vi "Folder Hierarchy to Tree.vi"(6 "Pattern":string, 8 "error in (no error)":errorcluster, 9 "Continue Recursing on Error? (F)":bool, 11 "File Explorer in":refnum<class "File Explorer.lvclass">) -> (0 "error out":errorcluster, 3 "File Explorer out":refnum<class "File Explorer.lvclass">)   [LabVIEW 2017, in "File Explorer.lvlib" / "File Explorer.lvclass"]
doc: "Parses the folder and harvests glyphs for each file type. Creates the tree items cluster for the tree control to render."
uses:
  <vilib>/gpm_packages/@cs/file-explorer-extension/Source/File Explorer/File Explorer/File Explorer.lvclass
  <vilib>/gpm_packages/@cs/file-explorer-extension/Source/File Explorer/File Explorer/File Explorer.lvclass/File Explorer.ctl
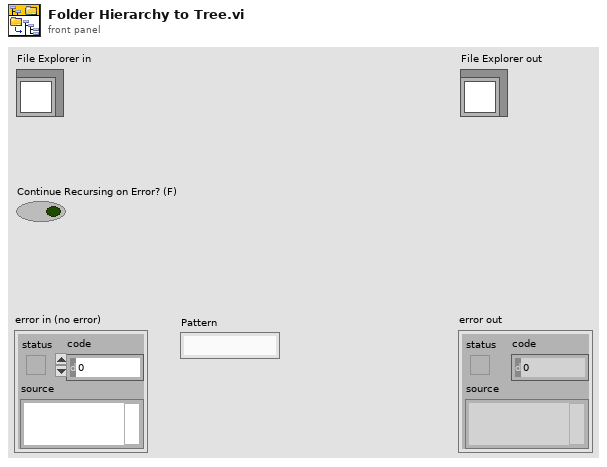
[diagram p1: front panel]
types:
  T1 = cluster{"Left Cell String":string, "Child Text":string[], "Child Tag":string, "Item Indent":i32, "Child Only?":bool, "Glyph Index":i32}
  T2 = typedef "imagedata.ctl" = cluster{"image type":i32, "image depth":i32, "image":u8[], "mask":u8[], "colors":u32[], "Rectangle":cluster{"left":i16, "top":i16, "right":i16, "bottom":i16}}
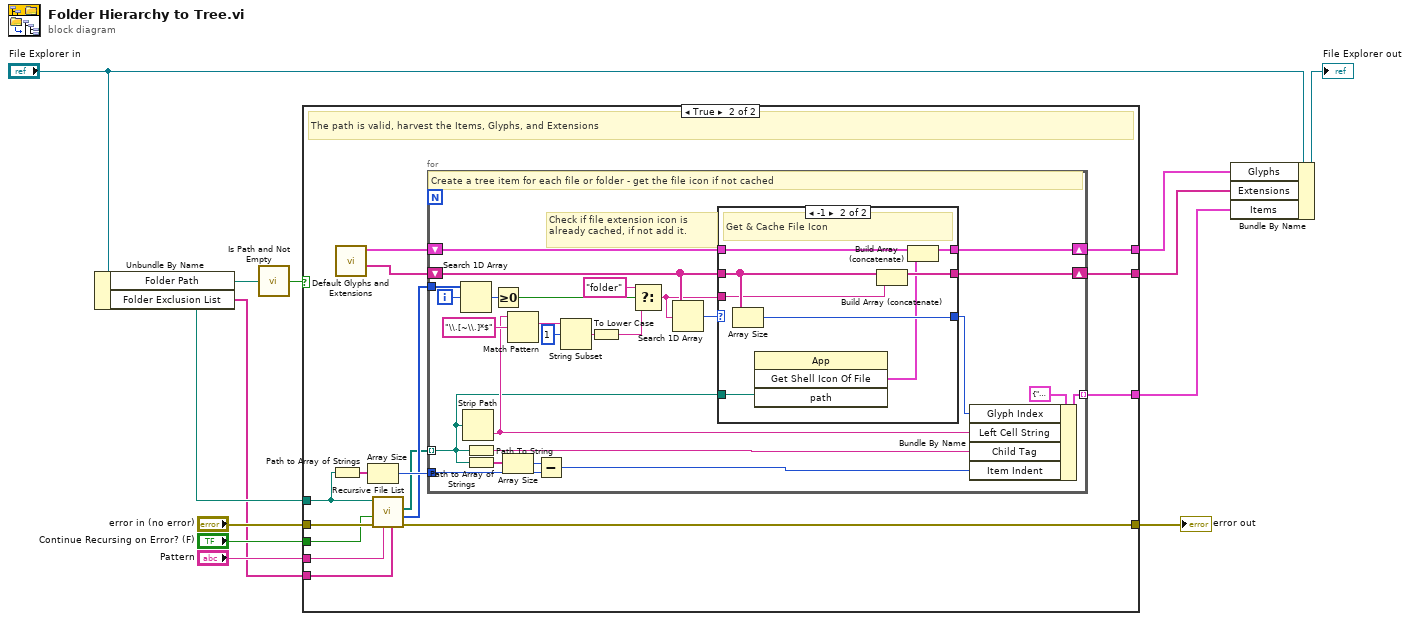
[diagram p0: block diagram]
diagram:
  n1 = Unbundle By Name("File Explorer in") -> ("Folder Path"=w7:path, "Folder Exclusion List"=w3:string[])
  n2 = call <vilib>:"Is Path and Not Empty.vi"("path"=w7) -> ("Is Path and Not Empty?"=w12:bool)  [unwired: 4 in]
  n3 = case shown="True" w12 {
    tunnel: w7 -> [_ w21]
    tunnel: [w13 w19] -> w10
    tunnel: "error in (no error)" -> [w13 w20]
    tunnel: "Continue Recursing on Error? (F)" -> [_ w16]
    tunnel: "Pattern" -> [_ w18]
    tunnel: w3 -> [_ w17]
    tunnel: [_ w26] -> w6
    tunnel: [_ w25] -> w5
    tunnel: [_ w24] -> w4
    frame False {
      # "The Path is either empty or Not a Path\nIn either case we will just ignore the request to recurse through the file hierarchy"
    }
    frame True {
      # "The path is valid, harvest the Items, Glyphs, and Extensions"
      n4 = Path to Array of Strings(0:w21) -> (2:w28:string[])  [unwired: 1 out]
      n5 = call <vilib>:"Default Glyphs and Extensions.vi"() -> ("Default Extensions"=w22:string[], "Default Glyphs"=w23:T2[])  [unwired: 10 in]
      n6 = Array Size(array=w28) -> (size(s)=w27:i32)
      n7 = call <vilib>:"Recursive File List.vi"("Folder to Exclude"=w17, "Pattern"=w18, "error in (no error)"=w20, "Continue Recursing on Error? (F)"=w16, "Folder Path"=w21) -> ("error out"=w19:errorcluster, "Folder Indexes"=w15:i32[], "Folders and Files"=w14:path[])  [unwired: 4 in]
      n8 = for {
        tunnel: w27 -> [w49]
        tunnel: w14 -> [w40] mode=indexing
        tunnel: [w48] -> w24 mode=indexing
        shift-right: [w37] -> w25
        shift-left: w22 -> [w36]
        shift-right: [w39] -> w26
        shift-left: w23 -> [w38]
        tunnel: w15 -> [w31]
        i -> [w32]
        # "Check if file extension icon is\nalready cached, if not add it."
        # "Create a tree item for each file or folder - get the file icon if not cached"
        n9 = Search 1D Array(1D array=w31, element=w32) -> (index of element=w30:i32)  [unwired: 1 in]
        n10 = Strip Path(path=w40) -> (name=w43:string)  [unwired: 1 out]
        n11 = Path To String(path=w40) -> (string=w53:string)
        n12 = Path to Array of Strings(0:w40) -> (2:w52:string[])  [unwired: 1 out]
        n13 = Greater Or Equal To 0?(x=w30) -> (x >= 0?=w29:bool)
        n14 = Array Size(array=w52) -> (size(s)=w51:i32)
        n15 = Match Pattern(string=w43, regular expression="\\.[~\\.]*$") -> (match substring=w44:string)  [unwired: 4 out]
        n16 = Subtract(x=w51, y=w49) -> (x-y=w50:i32)
        n17 = String Subset(string=w44, offset (0)=1) -> (substring=w45:string)  [unwired: 1 out]
        n18 = To Lower Case(string=w45) -> (all lower case string=w34:string)
        n19 = Select(t="folder", s=w29, f=w34) -> (s? t:f=w33:string)
        n20 = Search 1D Array(1D array=w36, element=w33) -> (index of element=w41:i32)  [unwired: 1 in]
        n21 = case shown="-1" w41 {
          selector: w41 -> [w55 _]
          tunnel: w40 -> [_ w65]
          tunnel: [w56 w59] -> w39
          tunnel: w38 -> [w56 w64]
          tunnel: [w57 w61] -> w37
          tunnel: w36 -> [w57 w63]
          tunnel: [w55 w62] -> w35
          tunnel: w33 -> [_ w60]
          frame Default {
            # "Glyph Found"
          }
          frame -1 {
            # "Get & Cache File Icon"
            n22 = Array Size(array=w63) -> (size(s)=w62:i32)
            n23 = invoke class="App" method="Get Shell Icon Of File"("path"=w65) -> ("GetShellIconOfFile"=w58:T2)  [unwired: 3 in, 3 out]
            n24 = Build Array (concatenate)(w63, w60) -> (w61:string[])
            n25 = Build Array (concatenate)(w64, w58) -> (w59:T2[])
          }
        }
        n26 = Bundle By Name(cluster=T1 {"Left Cell String"="", "Child Text"=[], "Child Tag"="", "Item Indent"=0, "Child Only?"=FALSE, "Glyph Index"=0} ("Item"), "Glyph Index"=w35, "Left Cell String"=w43, "Child Tag"=w53, "Item Indent"=w50) -> (w48:T1)
      }
    }
  }
  "error out" <- w10
  n27 = Bundle By Name(cluster="File Explorer in", "Glyphs"=w6, "Extensions"=w5, "Items"=w4) -> (→"File Explorer out":refnum<class "File Explorer.lvclass">)
